vi "GUID_LicencePath_write_in_editVI.vi"(8 "error in (no error)":errorcluster, 9 "LicencePath":path, 11 "GUID_Edit_path":path) -> (0 "error out":errorcluster)   [LabVIEW 2018]
uses:
  <vilib>/Utility/config.llb/Write Key (String).vi
  <vilib>/Utility/config.llb/NI_LVConfig.lvlib
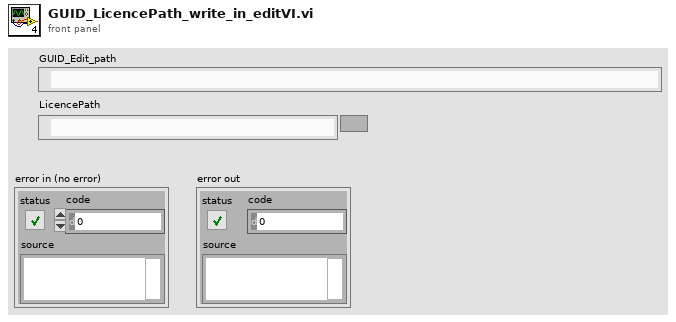
[diagram p1: front panel]
types:
  T1 = typedef "NI_LVConfig.lvlib/Config Data RefNum.ctl" = refnum<k1>
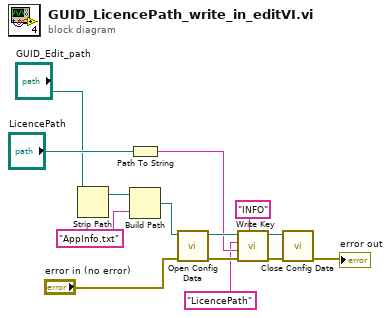
[diagram p0: block diagram]
diagram:
  n1 = Strip Path(path="GUID_Edit_path") -> (stripped path=w12:path)  [unwired: 1 out]
  n2 = Path To String(path="LicencePath") -> (string=w7:string)
  n3 = Build Path(base path=w12, name or relative path="AppInfo.txt") -> (appended path=w10:path)
  n4 = call <vilib>:"Open Config Data.vi"("error in (no error)"="error in (no error)", "configuration file path"=w10) -> ("error out"=w9:errorcluster, "refnum"=w8:T1)  [unwired: 7 in, 1 out]
  n5 = call-poly <vilib>:"Write Key.vi"("section"="INFO", "error in (no error)"=w9, "value"=w7, "key"="LicencePath", "refnum"=w8) -> ("error out"=w4:errorcluster, "refnum out"=w3:T1)  [unwired: 4 in, 1 out]
  n6 = call <vilib>:"Close Config Data.vi"("error in (no error)"=w4, "refnum"=w3) -> ("error out"=→"error out":errorcluster)  [unwired: 8 in, 1 out]
